vi "ex1_snap.vi"() -> ()   [LabVIEW 2012]
panel:
  out "error status":errorcluster
  out "Preview Window":picture
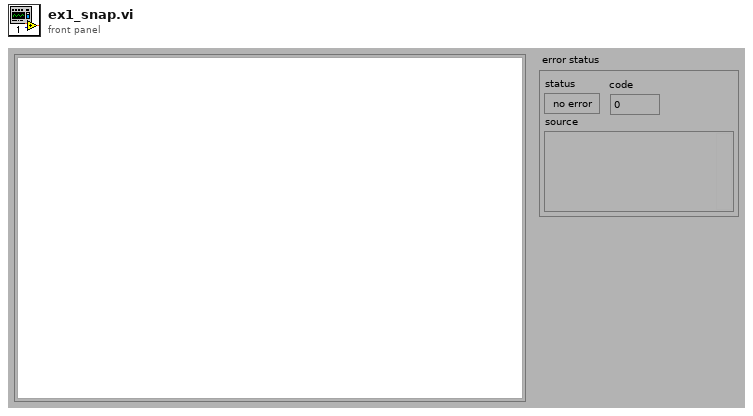
[diagram p1: front panel]
types:
  T1 = typedef "IMAQ Image.ctl" = refnum<image>
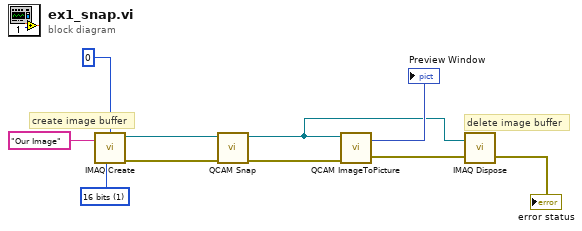
[diagram p0: block diagram]
diagram:
  w10 = u32 1 items=["8 bits", "16 bits"] ("Image Type")
  # "create image buffer"
  # "delete image buffer"
  n1 = call "IMAQ Create"("Border Size"=0, "Image Name"="Our Image", "Image Type"=w10) -> ("New Image"=w8:T1, "error out"=w5:errorcluster)  [unwired: 1 in, 1 out]
  n2 = call <userlib>:"QCAM Snap.vi"("error in (no error)"=w5, "New Image"=w8) -> ("error out"=w6:errorcluster, "Image Out"=w3:T1)  [unwired: 3 in, 5 out]
  n3 = call <userlib>:"QCAM ImageToPicture.vi"("error in (no error)"=w6, "Image"=w3) -> ("error out"=w7:errorcluster, "Picture Out"=→"Preview Window":picture)
  n4 = call "IMAQ Dispose"("Image"=w3, "error in (no error)"=w7) -> ("error out"=→"error status":errorcluster)  [unwired: 1 in, 3 out]
